vi "Untitled 1.vi"() -> ()   [LabVIEW 2020]
uses:
  <userlib>/_OpenG.lib/array/array.llb/Search 1D Array (Boolean)__ogtk.vi
  <userlib>/_OpenG.lib/array/array.llb/Index 1D Array Elements (String)__ogtk.vi
panel:
  out "elements":string[](array[string])
  out "array 2":string[](array[string])
  out "x = y?":bool[](array[boolean])
  out "spreadsheet string 2":string
  out "array":string[](array[string])
  out "spreadsheet string":string
  out "subarray":string[](array[string])
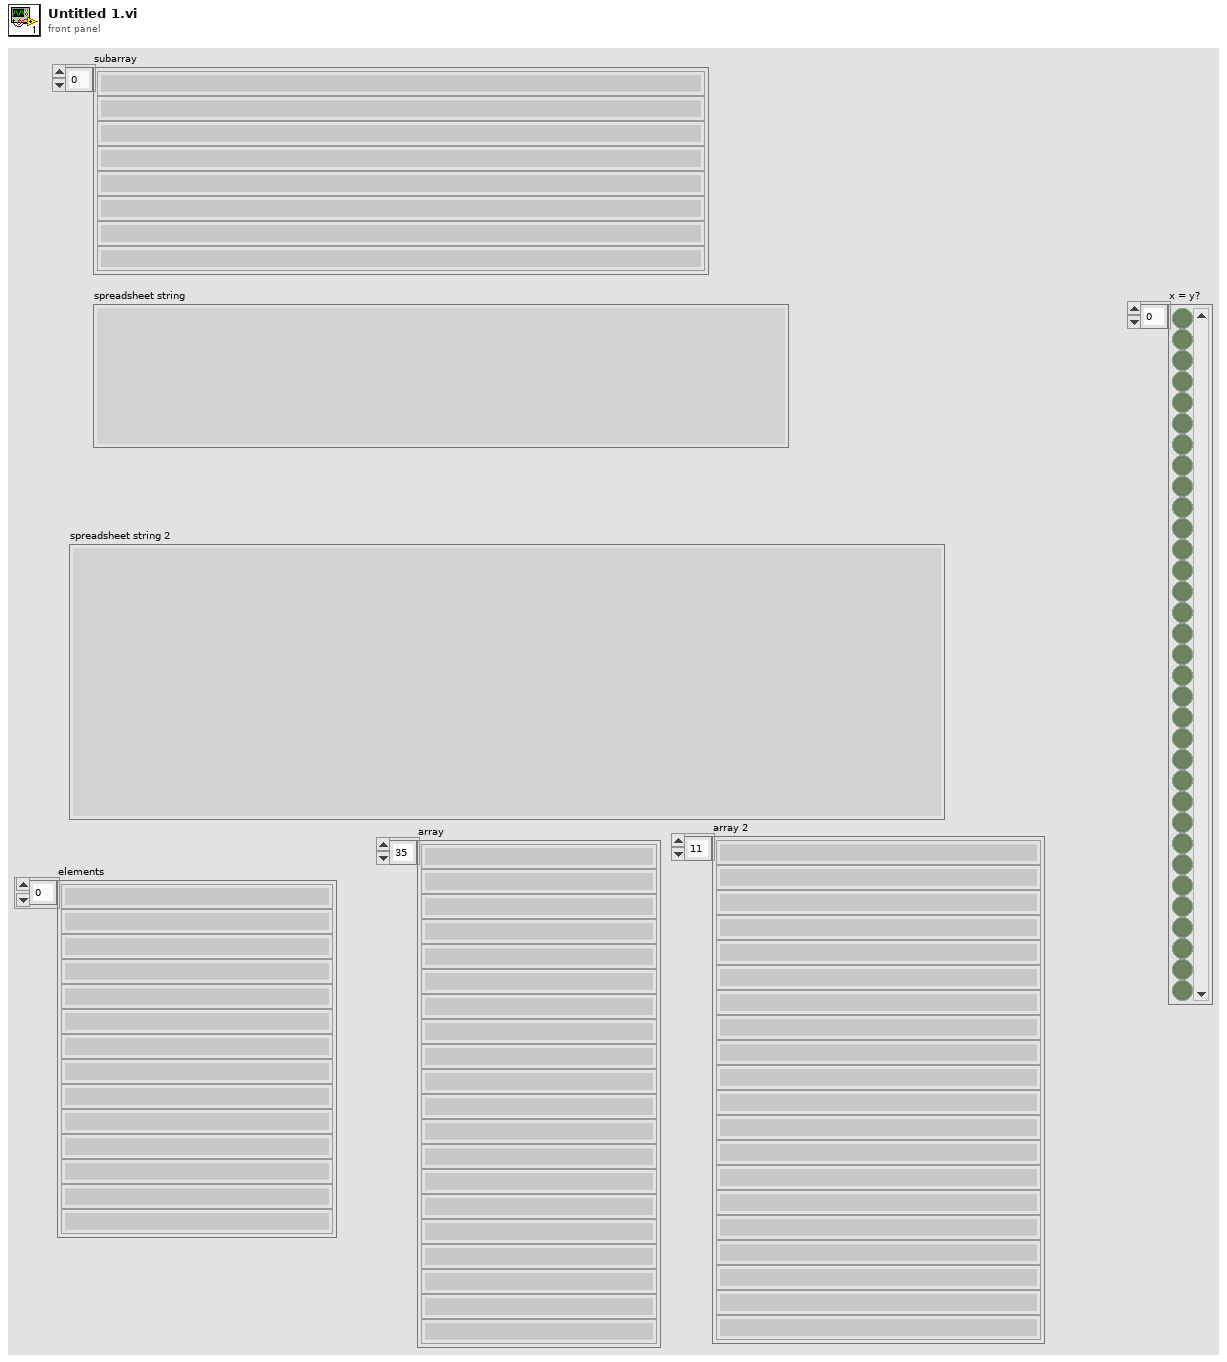
[diagram p1: front panel]
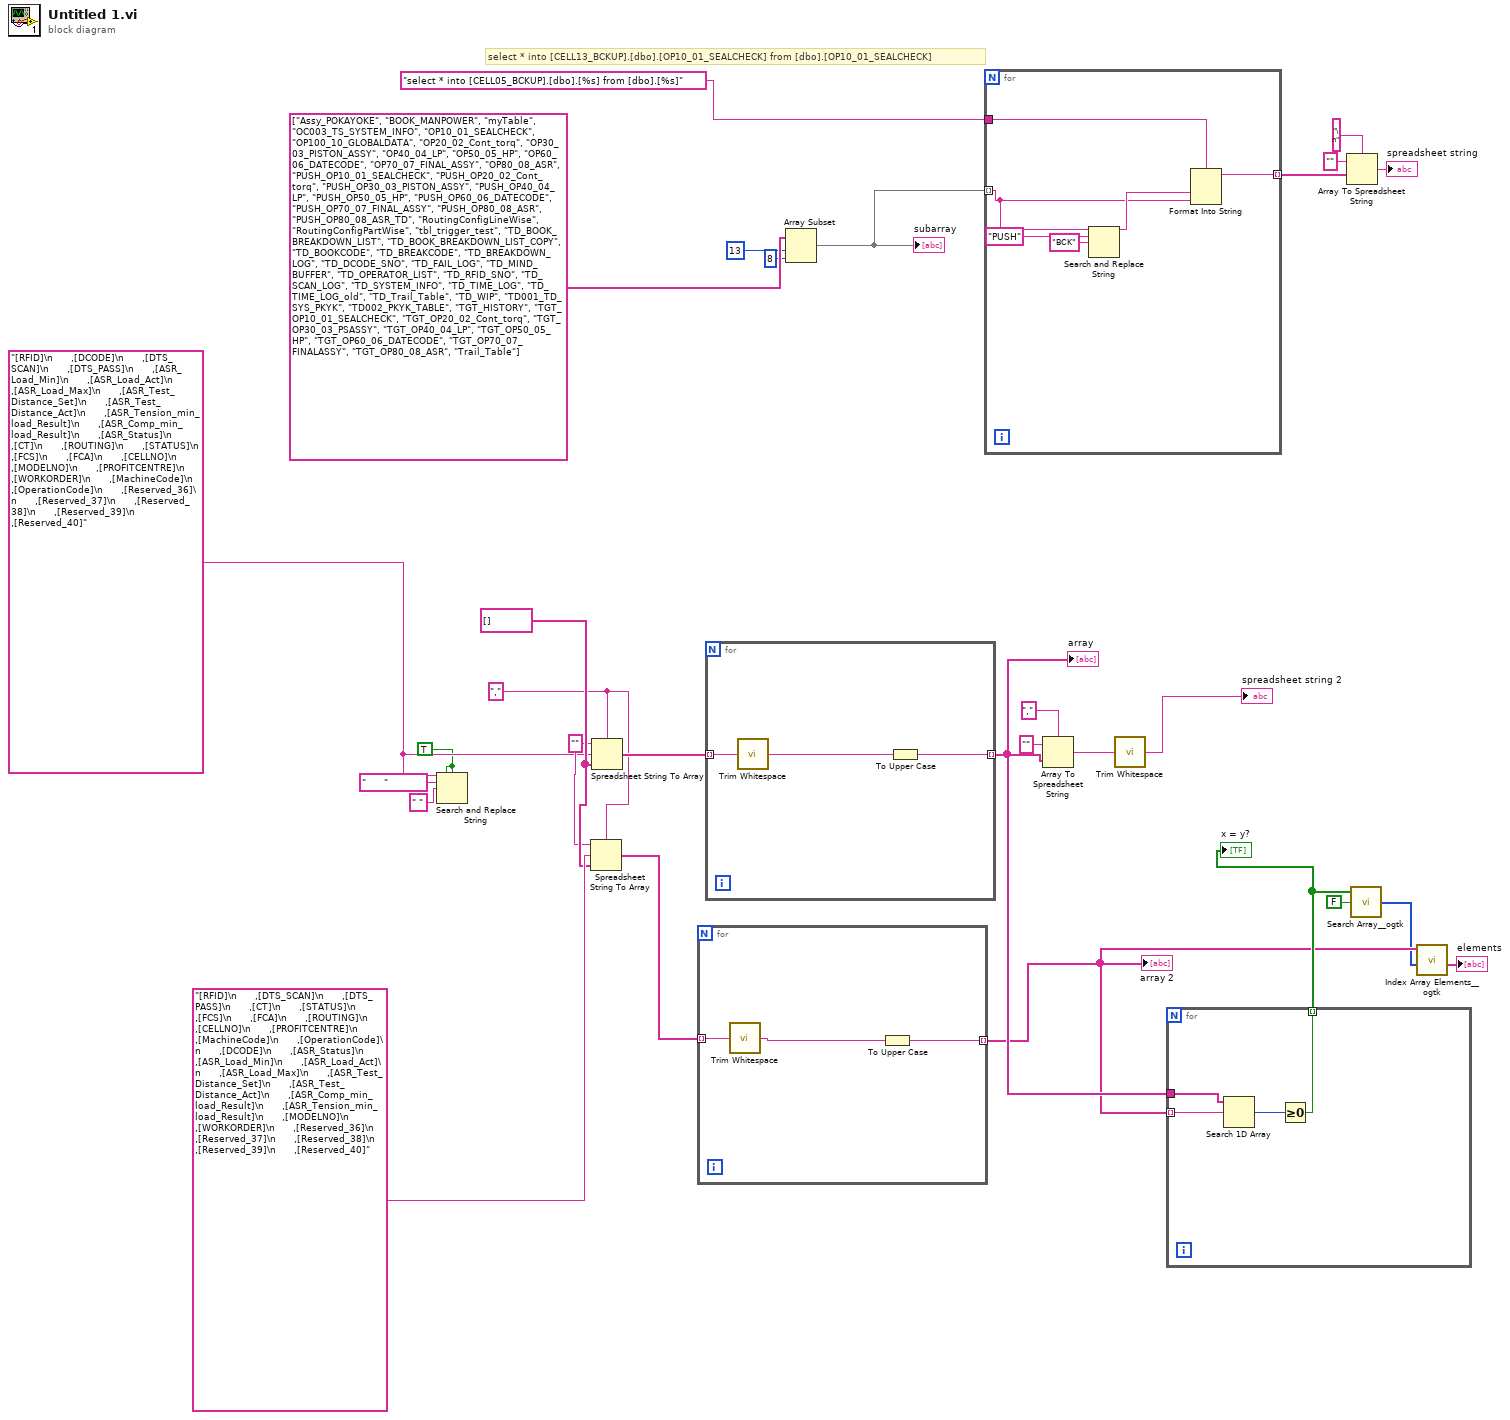
[diagram p0: block diagram]
diagram:
  w7 = TRUE ("ignore case? (F)")
  w13 = "," ("delimiter (Tab)")
  w14 = "" ("format string")
  w15 = string[] [] ("tables")
  w10 = "[RFID]\n      ,[DCODE]\n      ,[DTS_SCAN]\n      ,[DTS_PASS]\n      ,[ASR_Load_Min]\n      ,[ASR_Load_Act]\n      ,[ASR_Load_Max]\n      ,[ASR_Test_Distance_Set]\n      ,[ASR_Test_Distance_Act]\n      ,[ASR_Tension_min_load_Result]\n      ,[ASR_Comp_min_load_Result]\n      ,[ASR_Status]\n      ,[CT]\n      ,[ROUTING]\n      ,[STATUS]\n      ,[FCS]\n      ,[FCA]\n      ,[CELLNO]\n      ,[MODELNO]\n      ,[PROFITCENTRE]\n      ,[WORKORDER]\n      ,[MachineCode]\n      ,[OperationCode]\n      ,[Reserved_36]\n      ,[Reserved_37]\n      ,[Reserved_38]\n      ,[Reserved_39]\n      ,[Reserved_40]" ("search string")
  # "select * into [CELL13_BCKUP].[dbo].[OP10_01_SEALCHECK] from [dbo].[OP10_01_SEALCHECK]"
  n1 = Search and Replace String(replace all?=w7, case sensitive?=w7, input string=w10, search string="      ", replace string=" " ("search string")) -> ()  [unwired: 3 in, 4 out]
  n2 = Spreadsheet String To Array(delimiter (Tab)=w13, format string=w14, spreadsheet string="[RFID]\n      ,[DTS_SCAN]\n      ,[DTS_PASS]\n      ,[CT]\n      ,[STATUS]\n      ,[FCS]\n      ,[FCA]\n      ,[ROUTING]\n      ,[CELLNO]\n      ,[PROFITCENTRE]\n      ,[MachineCode]\n      ,[OperationCode]\n      ,[DCODE]\n      ,[ASR_Status]\n      ,[ASR_Load_Min]\n      ,[ASR_Load_Act]\n      ,[ASR_Load_Max]\n      ,[ASR_Test_Distance_Set]\n      ,[ASR_Test_Distance_Act]\n      ,[ASR_Comp_min_load_Result]\n      ,[ASR_Tension_min_load_Result]\n      ,[MODELNO]\n      ,[WORKORDER]\n      ,[Reserved_36]\n      ,[Reserved_37]\n      ,[Reserved_38]\n      ,[Reserved_39]\n      ,[Reserved_40]" ("search string"), array type (2D Dbl)=w15) -> (array=w12:string[])
  n3 = Spreadsheet String To Array(delimiter (Tab)=w13, format string=w14, spreadsheet string=w10, array type (2D Dbl)=w15) -> (array=w20:string[])
  n4 = for {
    tunnel: w12 -> [w32] mode=indexing
    tunnel: [w30] -> w4 mode=indexing
    n5 = call <vilib>:"Trim Whitespace.vi"("string"=w32) -> ("trimmed string"=w31:string)  [unwired: 1 in]
    n6 = To Upper Case(1:w31) -> (0:w30:string)
  }
  "array 2" <- w4
  n7 = for {
    tunnel: w20 -> [w35] mode=indexing
    tunnel: [w33] -> w11 mode=indexing
    n8 = call <vilib>:"Trim Whitespace.vi"("string"=w35) -> ("trimmed string"=w34:string)  [unwired: 1 in]
    n9 = To Upper Case(1:w34) -> (0:w33:string)
  }
  "array" <- w11
  n10 = Array Subset(array=string[] ["Assy_POKAYOKE", "BOOK_MANPOWER", "myTable", "OC003_TS_SYSTEM_INFO", "OP10_01_SEALCHECK", "OP100_10_GLOBALDATA", "OP20_02_Cont_torq", "OP30_03_PISTON_ASSY", "OP40_04_LP", "OP50_05_HP", "OP60_06_DATECODE", "OP70_07_FINAL_ASSY", "OP80_08_ASR", "PUSH_OP10_01_SEALCHECK", "PUSH_OP20_02_Cont_torq", "PUSH_OP30_03_PISTON_ASSY", "PUSH_OP40_04_LP", "PUSH_OP50_05_HP", "PUSH_OP60_06_DATECODE", "PUSH_OP70_07_FINAL_ASSY", "PUSH_OP80_08_ASR", "PUSH_OP80_08_ASR_TD", "RoutingConfigLineWise", "RoutingConfigPartWise", "tbl_trigger_test", "TD_BOOK_BREAKDOWN_LIST", "TD_BOOK_BREAKDOWN_LIST_COPY", "TD_BOOKCODE", "TD_BREAKCODE", "TD_BREAKDOWN_LOG", "TD_DCODE_SNO", "TD_FAIL_LOG", "TD_MIND_BUFFER", "TD_OPERATOR_LIST", "TD_RFID_SNO", "TD_SCAN_LOG", "TD_SYSTEM_INFO", "TD_TIME_LOG", "TD_TIME_LOG_old", "TD_Trail_Table", "TD_WIP", "TD001_TD_SYS_PKYK", "TD002_PKYK_TABLE", "TGT_HISTORY", "TGT_OP10_01_SEALCHECK", "TGT_OP20_02_Cont_torq", "TGT_OP30_03_PSASSY", "TGT_OP40_04_LP", "TGT_OP50_05_HP", "TGT_OP60_06_DATECODE", "TGT_OP70_07_FINALASSY", "TGT_OP80_08_ASR", "Trail_Table"] ("tables"), index=13, length=8) -> (w26:string[])
  "subarray" <- w26
  n11 = for {
    tunnel: w26 -> [w37] mode=indexing
    tunnel: "select * into [CELL05_BCKUP].[dbo].[%s] from [dbo].[%s]" ("String") -> [w41]
    tunnel: [w36] -> w24 mode=indexing
    n12 = Search and Replace String(input string=w37, search string="PUSH", replace string="BCK" ("replace string (\"\")")) -> (result string=w38:string)  [unwired: 5 in, 3 out]
    n13 = Format Into String(format string=w41, w38, w37) -> (resulting string=w36:string)  [unwired: 2 in, 1 out]
  }
  n14 = Array To Spreadsheet String(delimiter (Tab)=",", array=w11, 3:"" ("format string")) -> (spreadsheet string=w17:string)
  n15 = call <vilib>:"Trim Whitespace.vi"("string"=w17) -> ("trimmed string"=→"spreadsheet string 2":string)  [unwired: 1 in]
  n16 = for {
    tunnel: w11 -> [w45]
    tunnel: w4 -> [w44] mode=indexing
    tunnel: [w42] -> w6 mode=indexing
    n17 = Search 1D Array(1D array=w45, element=w44) -> (index of element=w43:i32)  [unwired: 1 in]
    n18 = Greater Or Equal To 0?(x=w43) -> (x >= 0?=w42:bool)
  }
  "x = y?" <- w6
  n19 = Array To Spreadsheet String(delimiter (Tab)="\n", array=w24, 3:"" ("format string")) -> (spreadsheet string=→"spreadsheet string":string)
  n20 = call-poly <userlib>:"Search Array__ogtk.vi"("Array"=w6, "Element Data"=FALSE) -> ("Indices of Elements"=w3:i32[])  [unwired: 7 in]
  n21 = call-poly <userlib>:"Index Array Elements__ogtk.vi"("indices"=w3, "array"=w4) -> ("elements"=→"elements":string[])  [unwired: 9 in]
